vi "Write Altura.vi"(8 "error in (no error)":errorcluster, 10 "Altura":dbl, 11 "Triangulo in":refnum<class "Triangulo.lvclass">) -> (0 "error out":errorcluster, 3 "Triangulo out":refnum<class "Triangulo.lvclass">)   [LabVIEW 2024, in "Triangulo.lvclass"]
uses:
  Triangulo.lvclass
  Triangulo.lvclass/Triangulo.ctl
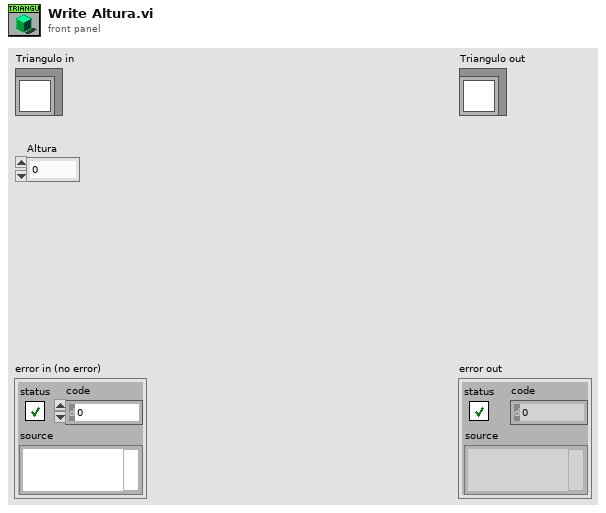
[diagram p1: front panel]
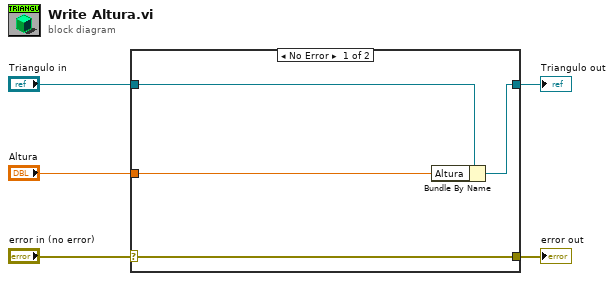
[diagram p0: block diagram]
diagram:
  n1 = case shown="No Error" "error in (no error)" {
    selector: "error in (no error)" -> [w9 w10]
    tunnel: [w9 w10] -> w4
    tunnel: [w7 w11] -> w2
    tunnel: "Triangulo in" -> [w8 w11]
    tunnel: "Altura" -> [w6 _]
    frame No Error {
      n2 = Bundle By Name(cluster=w8, "Altura"=w6) -> (w7:refnum<class "Triangulo.lvclass">)
    }
    frame Error {
    }
  }
  "error out" <- w4
  "Triangulo out" <- w2
